vi "Drag Panel-Move Window.vi"(8 "error in":errorcluster, 11 "Window ID":u32) -> (0 "error out":errorcluster)   [LabVIEW 2018]
uses:
  USER32.DLL
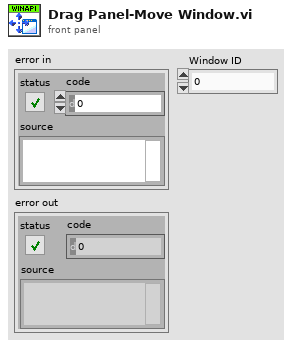
[diagram p1: front panel]
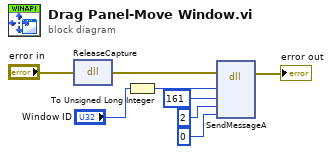
[diagram p0: block diagram]
diagram:
  n1 = dll-call lib="user32.dll" fn="ReleaseCapture"(error in="error in") -> (error out=w2:errorcluster)  [unwired: 3 in, 1 out]
  n2 = To Unsigned Long Integer(number="Window ID") -> (unsigned 32bit integer=w4:u32)
  n3 = dll-call lib="user32.dll" fn="SendMessageA"(error in=w2, "hWnd"=w4, "Msg"=161, "wParam"=2, "lParam"=0) -> (error out=→"error out":errorcluster)  [unwired: 7 in, 1 out]
